vi "acquire_image_pixelfly.vi"(0 "boardid":i32, 1 "Buffer address":i32, 2 "Array input":u16[][](array[numeric]), 3 "error in":errorcluster, 5 "Size":i32, 6 "Buffer number":i32) -> (4 "Buffer status":T1, 7 "image array":dbl[][](array[numeric]), 8 "error out":errorcluster)   [LabVIEW 2013]
doc: "Take a single PixelFly exposure and display the result as an intensity graph.This VI illustrates the basics of taking an exposure with the PixelFly camera. Use Ctrl-H to get help on any of the controls\n\nCopyright 2001, The Cooke Corporation."
panel:
  # "Take a single PixelFly exposure and display the result as an intensity graph."
  # "This VI illustrates the basics of taking an exposure with the PixelFly camera. Use Ctrl-H to get help on any of the controls\n\nCopyright 2001, The Cooke Corporation."
  # "Note that the image is inverted. The image reads out from top to bottom, but intensity graph plots bottom to top"
  # "Status flags"
  # "Buffer errors"
  # "Memory usage"
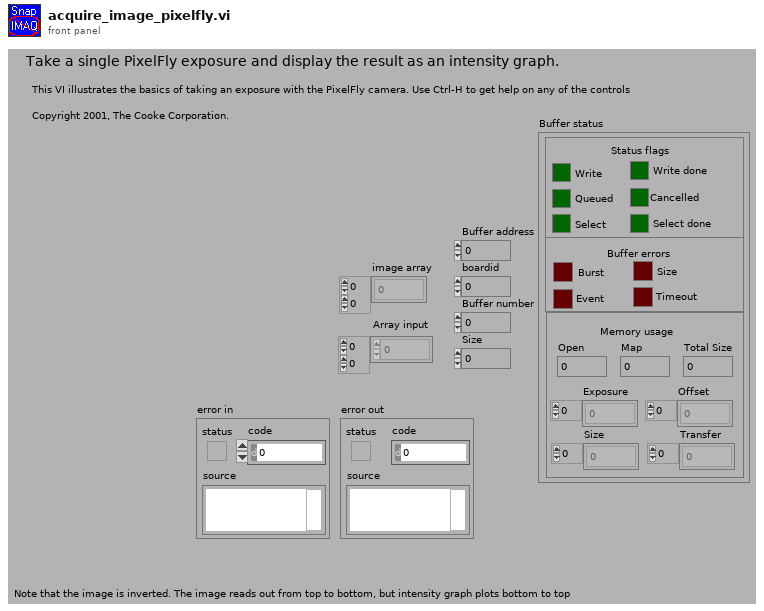
[diagram p1: front panel]
types:
  T1 = cluster{"Write":bool, "Write done":bool, "Queued":bool, "Cancelled":bool, "Select":bool, "Select done":bool, "Burst":bool, "Size":bool, "Event":bool, "Timeout":bool, "Open":i32, "Map":i32, "Exposure":i32[], "Offset":i32[], "Size":i32[], "Transfer":i32[], "Total Size":i32}
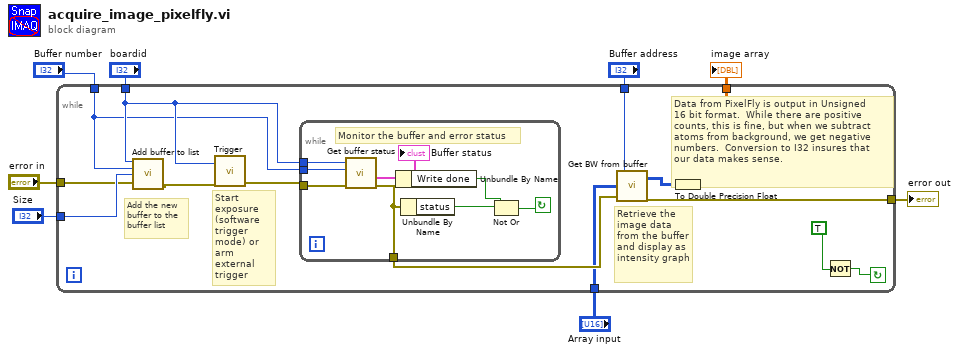
[diagram p0: block diagram]
diagram:
  n1 = while {
    tunnel: "error in" -> [w16]
    tunnel: "Buffer address" -> [w17]
    tunnel: "Array input" -> [w18]
    tunnel: [w19] -> w3
    tunnel: "Size" -> [w21]
    tunnel: "boardid" -> [w14]
    tunnel: "Buffer number" -> [w13]
    tunnel: [w9] -> w1
    stop <- w12 continue-if-true
    # "Data from PixelFly is output in Unsigned\n16 bit format.  While there are positive\ncounts, this is fine, but when we subtract \natoms from background, we get negative\nnumbers.  Conversion to I32 insures that\nour data makes sense."
    # "Retrieve the image data from the buffer and display as intensity graph"
    # "Start exposure (software trigger mode) or arm external trigger"
    # "Add the new buffer to the buffer list"
    n2 = call "Add buffer to list.vi"("Handle in"=w14, "Buffer in"=w13, "size"=w21, "error in (no error)"=w16) -> ("error out"=w15:errorcluster)  [unwired: 9 in, 2 out]
    n3 = call "Trigger.vi"("Handle in"=w14, "error in (no error)"=w15) -> ("error out"=w22:errorcluster)  [unwired: 2 out]
    n4 = while {
      tunnel: [w23] -> w20
      tunnel: w22 -> [w28]
      tunnel: w13 -> [w29]
      tunnel: w14 -> [w30]
      stop <- w24 continue-if-true
      # "Monitor the buffer and error status"
      n5 = call "Get buffer status.vi"("error in (no error)"=w28, "Buffer request"=w29, "Handle in"=w30) -> ("error out"=w23:errorcluster, "Buffer status"=w27:T1)  [unwired: 1 in, 2 out]
      "Buffer status" <- w27
      n6 = Unbundle By Name(w27) -> ("Write done"=w26:bool)
      n7 = Unbundle By Name(w23) -> ("status"=w25:bool)
      n8 = Not Or(1:w25, 2:w26) -> (0:w24:bool)
    }
    n9 = call "Get BW from buffer.vi"("error in (no error)"=w20, "Array input"=w18, "Buffer address"=w17) -> ("error out"=w19:errorcluster, "Image data"=w10:u16[][])
    n10 = To Double Precision Float(number=w10) -> (double precision float=w9:dbl[][])
    n11 = Not(x=TRUE ("stop 2")) -> (.not. x?=w12:bool)
  }
  "error out" <- w3
  "image array" <- w1
